vi "Example.vi"() -> ()   [LabVIEW 2020]
doc: "Demonstrate some of the aspect of the Firmata Protocol."
uses:
  FirmataClient/controls/PinModesListData.ctl
  FirmataClient/controls/PinModeData.ctl
  FirmataClient/controls/FirmataPinModes.ctl
  FirmataClient/controls/FGV-Mode.ctl
  FirmataClient.lvlib
panel:
  in  "Display Numbers As Decimal":bool
  in  "Send":bool
  in  "Stop":bool
  in  "Tab Control":T1(tab)
  out "Firmata Firmware Version GF":string caption="Firmata Firmware Version"
  out "Firmata Firmware Name GF":string caption="Firmata Firmware Name"
  out "IsValidSysex":bool
  out "FirmataFirmwareVersion":string
  out "IsValidReply":bool
  out "IsValidSysex 2":bool caption="IsValidSysex"
  out "Board Pins":T2[](array[typedef]) {"Index"."DigitalIndex" step=1 format="D%d"; "Index"."AnalogIndex" min=0.0 step=1.0 format="A%#.0g"}
  in  "Enable Reporting? SAPR":bool caption="Enable Reporting?"
  in  "Pin Index SAPR":u8 caption="Pin Index" format="%.0x"
  out "AnalogADCValues":u16[](array[numeric])
  in  "Pin Index GPS 2":u8 caption="Pin Index" format="%.0x"
  out "Pin Index GPS":u8 caption="Pin Index" format="%.0x"
  out "Pin State GPS":u64 caption="Pin State" format="%.0x"
  out "Pin Mode GPS":T4=enum."Extended.DHT" caption="Pin Mode"
  out "Analog Mappings":dbl[](array[numeric])
  in  "Enable Reporting?":bool
  in  "Port Index SDPR":u8 caption="Port Index" format="%.0x"
  out "PortValue":u16 format="%.0x"
  out "PortValueAsArray":bool[](array[boolean])
  out "Port Index 2":u8 format="%.0x"
  in  "Pin Index SPM":u8 caption="Pin Index" format="%.0x"
  in  "Pin Mode":T4
  in  "Pin State":bool
  in  "Pin Index SDP":u8 caption="Pin Index" format="%.0x"
  in  "Pin Value":u16 format="%.0x"
  in  "Pin Index":u8 format="%.0x"
  in  "Port State":bool[](array[boolean])
  in  "Port Index":u8 format="%.0x"
  in  "comport":refnum<visa-resource-name>="COM20"
  in  "baud rate":u32=57600
  out "Messages":string
  # "Set Board Comport and Baud Rate, Run the VI.\nWhen initialization is successful, select tab, read instructions and click on send.\n\nThis is a partial implementation of the Firmata protocol.\nFor more information, https://github.com/firmata/protocol/blob/master/protocol.md#message-types"
  # "Get the remote device/microcontroller to reset.\n\nClick on the \"Send Message\" button."
  # "Obtain the name of the sketch running on the remote device/microcontroller along with its version.\n\nClick on the \"Send Message\" button."
  # "Obtain the version of the sketch running on the remote device/microcontroller.\n\nClick on the \"Send Message\" button."
  # "In reporting mode, the remote device/microcontroller puts a message on the serial line everytime the value of the (input) line being reported on changes.\n\nPins are numbered from 0 to the total number of IO lines the microcontroller supports. One must then make sure to find the offset/index for the line.\n\nSet an index for the line to use,\nSet reporting to true or false.\n\nClick on the \"Send Message\" button."
  # "In reporting mode, the remote device/microcontroller puts a message on the serial line everytime the value of the (input) line being reported on changes.\n\nPins are numbered from 0 to the total number of IO lines the microcontroller supports. One must then make sure to find the offset/index for the line.\n\nSet an index for the line to use,\nSet reporting to true or false.\n\nClick on the \"Send Message\" button."
  # "In reporting mode, the remote device/microcontroller puts a message on the serial line everytime the value of the (input) line being reported on changes.\n\nPins are numbered from 0 to the total number of IO lines the microcontroller supports. One must then make sure to find the offset/index for the line.\n\nSet an index for the line to use,\nSet reporting to true or false.\n\nClick on the \"Send Message\" button."
  # "In reporting mode, the remote device/microcontroller puts a message on the serial line everytime the value of the (input) line being reported on changes.\n\nPins are numbered from 0 to the total number of IO lines the microcontroller supports. One must then make sure to find the offset/index for the line.\n\nSet an index for the line to use,\nSet reporting to true or false.\n\nClick on the \"Send Message\" button."
  # "The firmata protocol allows control of pin under various modes (digital input, output, analog input, pwm,...)\n\nPins are numbered from 0 to the total number of IO lines the microcontroller supports. One must then make sure to find the offset/index for the line.\n\nSet an index for the line to use,\nSet line new mode.\n\nClick on the \"Send Message\" button."
  # "In reporting mode, the remote device/microcontroller puts a message on the serial line everytime the value of the line being reported on changes.\n\nPins are numbered from 0 to the total number of IO lines the microcontroller supports. One must then make sure to find the offset/index for the line.\n\nSet an index for the line to use,\nSet reporting to true or false.\n\nClick on the \"Send Message\" button."
  # "An Analog message can convey the current value on the line or, if the line is configured as an analog output, the value for the DAC can be passed along. Typically this value is a 14bits value depending on the resolution of the pin\n\nPins are numbered from 0 to the total number of IO lines the microcontroller supports. One must then make sure to find the offset/index for the line.\n\nSet an index for the line to use,\nSet line value.\n\nClick on the \"Send Message\" button."
  # "Available pins are logically divided in ports of 8 bits each. Given the index of the pins to control, compute the index of the port (pinIndex / 8), and the offset of the pin within the port (pinIndex % 8) and set the required value.\n\nSet an index for the port to use,\nSet line states.\n\nClick on the \"Send Message\" button."
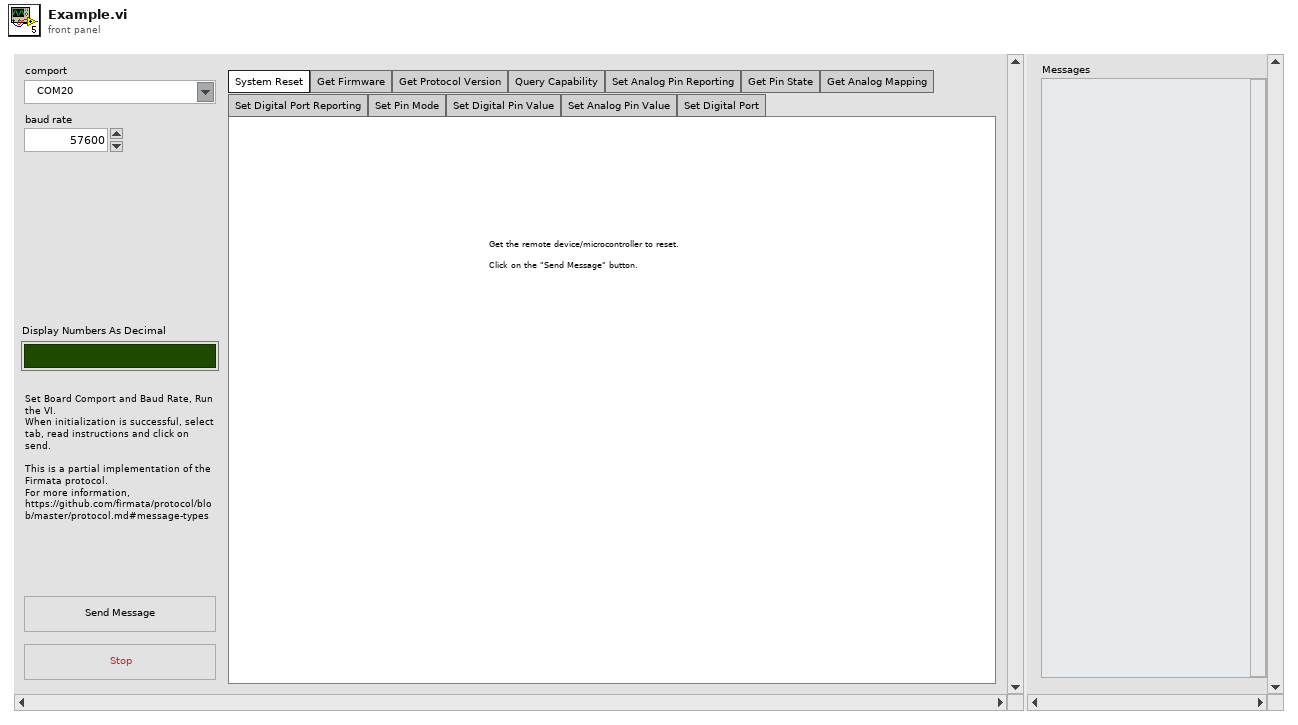
[diagram p1: front panel]
types:
  T1 = enum32{"System Reset", "Get Firmware", "Get Protocol Version", "Query Capability", "Set Analog Pin Reporting", "Get Pin State", "Get Analog Mapping", "Set Digital Port Reporting", "Set Pin Mode", "Set Digital Pin Value", "Set Analog Pin Value", "Set Digital Port"}
  T2 = typedef "FirmataClient.lvlib/PinModesListData.ctl" = cluster{"DigitalInputMode":T3, "DigitalOutputMode":T3, "AnalogInputMode":T3, "PWMMode":T3, "ServoMode":T3, "ShiftMode":T3, "I2CMode":T3, "OneWireMode":T3, "StepperMode":T3, "EncoderMode":T3, "SerialMode":T3, "InputPullupMode":T3, "Ext.SPIMode":T3, "Ext.SonarMode":T3, "Ext.ToneMode":T3, "Ext.DHTMode":T3, "Index":cluster{"DigitalIndex":u16, "AnalogIndex":dbl}}
  T3 = typedef "FirmataClient.lvlib/PinModeData.ctl" = cluster{"Resolution":u8, "btn":bool, "PinMode":T4}
  T4 = typedef "FirmataClient.lvlib/FirmataPinModes.ctl" = enum16{"DigitalInput", "DigitalOutput", "AnalogInput", "PWM", "Servo", "Shift", "I2C", "OneWire", "Stepper", "Encoder", "Serial", "InputPullup", "Extended.SPI", "Extended.Sonar", "Extended.Tone", "Extended.DHT"}
  T5 = typedef "FirmataClient.lvlib/FGV-Mode.ctl" = enum16{"Load Comport", "Load Board Capabilities", "Read"}
  T6 = typedef "FirmataClient.lvlib/FirmataProtocolConstants.ctl" = u16
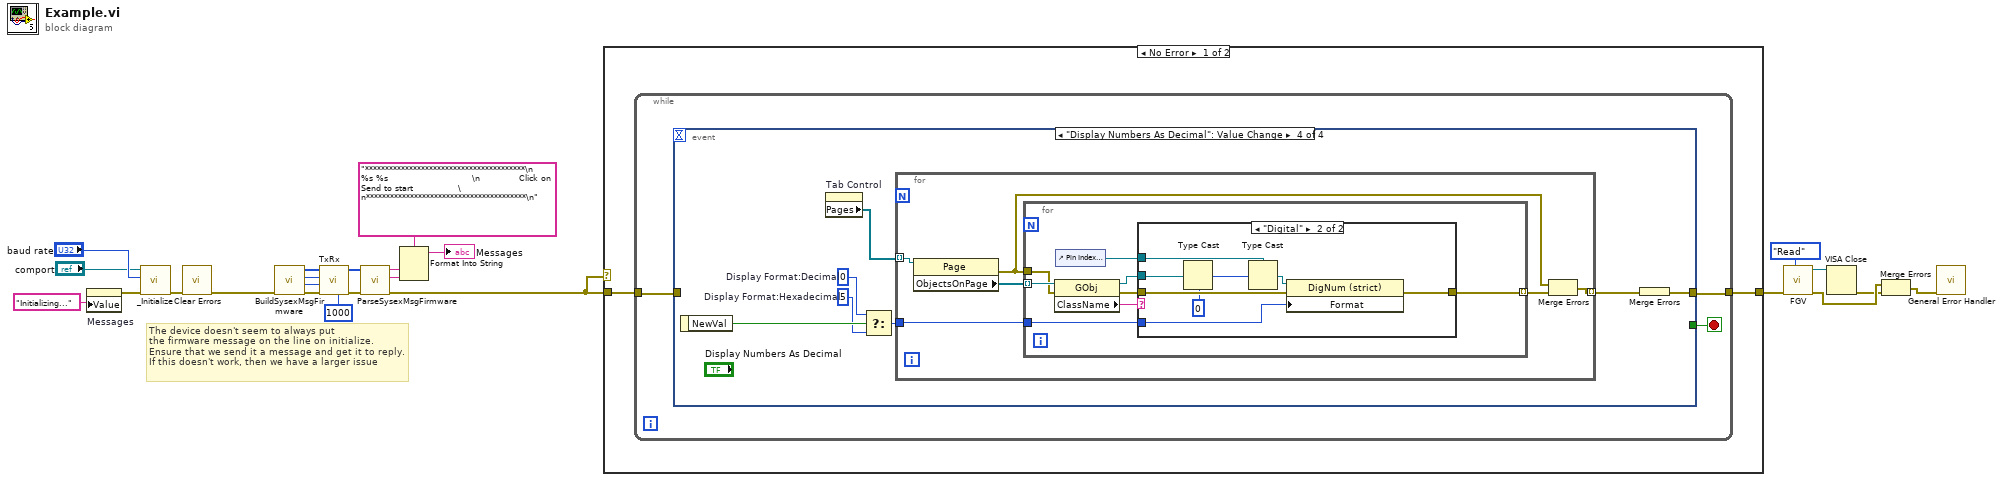
[diagram p0: block diagram]
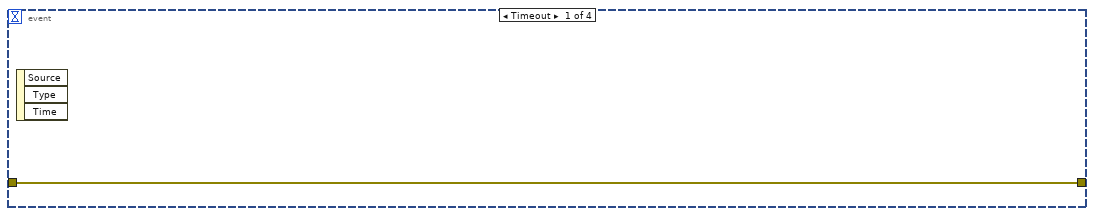
[diagram p2: hidden frame]
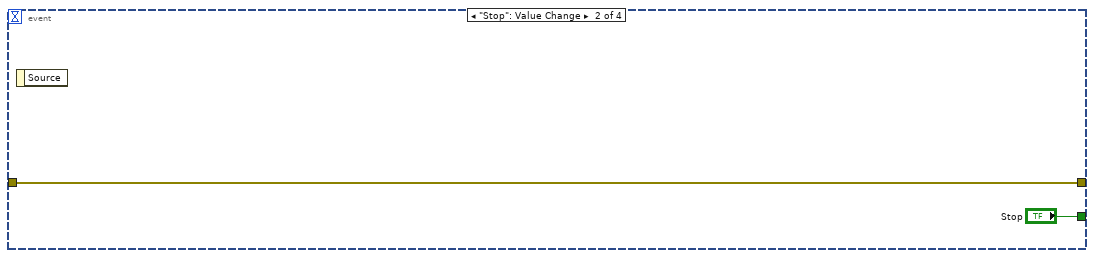
[diagram p3: hidden frame]
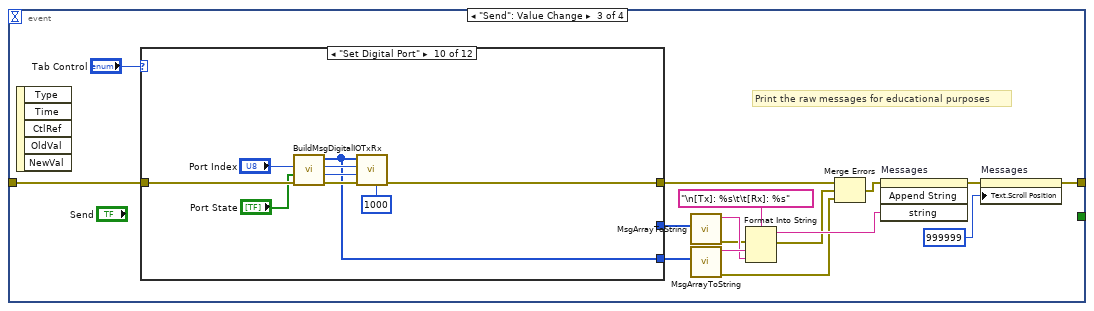
[diagram p4: hidden frame]
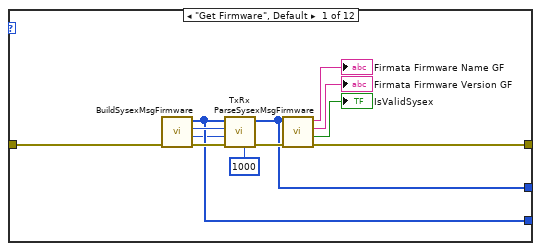
[diagram p5: hidden frame]
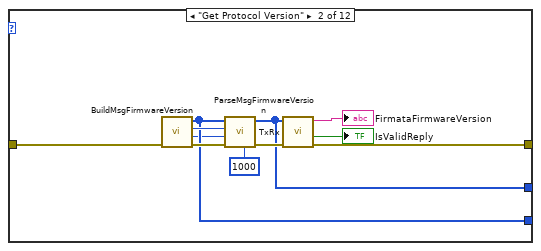
[diagram p6: hidden frame]
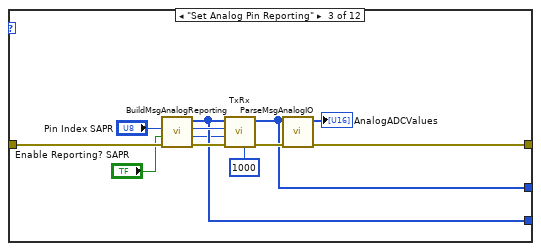
[diagram p7: hidden frame]
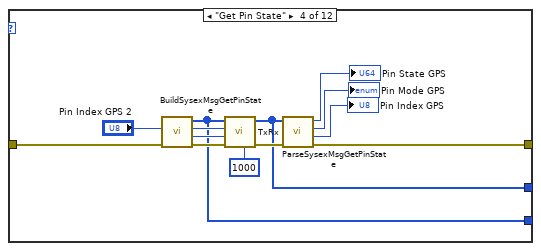
[diagram p8: hidden frame]
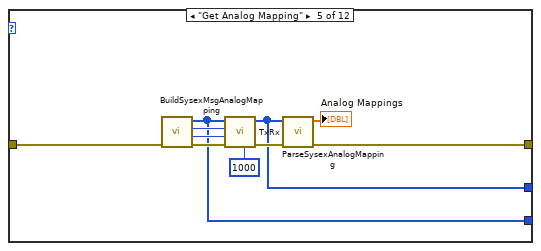
[diagram p9: hidden frame]
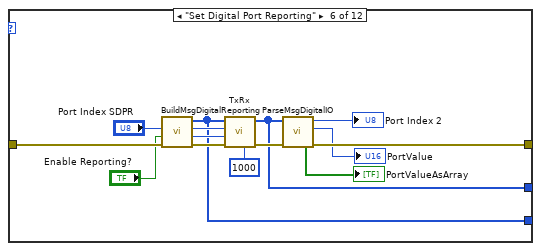
[diagram p10: hidden frame]
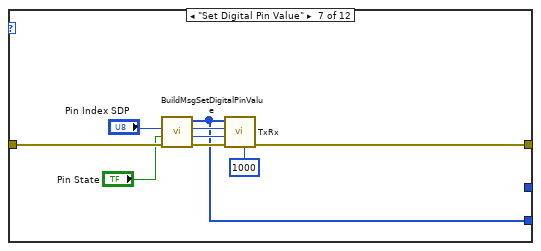
[diagram p11: hidden frame]
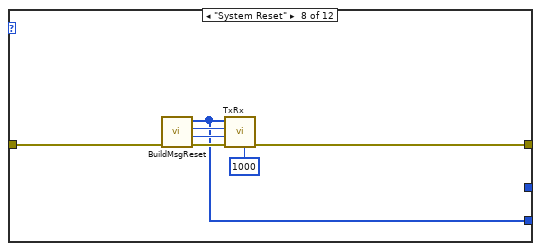
[diagram p12: hidden frame]
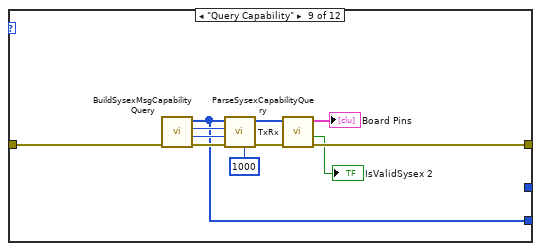
[diagram p13: hidden frame]
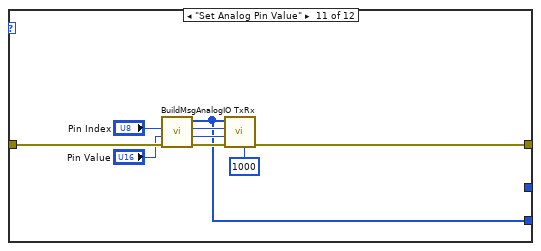
[diagram p14: hidden frame]
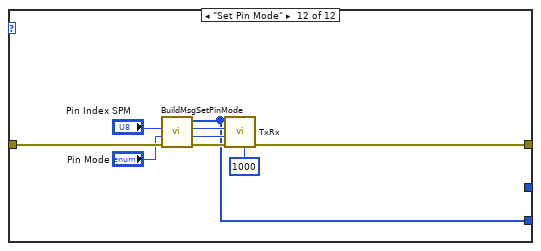
[diagram p15: hidden frame]
diagram:
  # "The device doesn't seem to always put \nthe firmware message on the line on initialize.\nEnsure that we send it a message and get it to reply.\nIf this doesn't work, then we have a larger issue"
  n1 = property on="Messages" class="Str"("Value"="Initializing..." ("Messages")) -> (error out=w19:errorcluster)  [unwired: 2 in, 1 out]
  n2 = call "_Initialize.vi"("error in"=w19, "baud rate"="baud rate", "comport"="comport") -> ("error out"=w15:errorcluster)  [unwired: 4 in, 4 out]
  n3 = call <vilib>:"Clear Errors.vi"("error in (no error)"=w15) -> ("error out"=w4:errorcluster)  [unwired: 5 in, 1 out]
  n4 = call "BuildSysexMsgFirmware.vi"("error in"=w4) -> ("error out"=w10:errorcluster, "ReplyLength"=w8:i32, "ReplyFirstByte"=w7:T6, "GetFirmwareMessage"=w6:u8[])  [unwired: 7 in]
  n5 = call "TxRx.vi"("Timeout"=u32 1000, "error in"=w10, "Expected Reply Length"=w8, "ReplyFirstByte"=w7, "MessageToSend"=w6) -> ("error out"=w11:errorcluster, "ReceivedMessage"=w5:u8[])  [unwired: 2 in, 3 out]
  n6 = call "ParseSysexMsgFirmware.vi"("error in"=w11, "Sysex Message"=w5) -> ("error out"=w3:errorcluster, "FirmataFirmwareVersion"=w2:string, "FirmataFirmwareName"=w1:string)  [unwired: 6 in, 1 out]
  n7 = Format Into String(format string="****************************************\n         %s %s                            \n             Click on Send to start               \n****************************************\n", w1, w2) -> (resulting string=→"Messages":string)  [unwired: 2 in, 1 out]
  n8 = case shown="No Error" w3 {
    tunnel: [w26 w204] -> w22
    tunnel: w3 -> [w25 w204]
    frame No Error {
      n9 = while {
        tunnel: [w28] -> w26
        tunnel: w25 -> [w27]
        stop <- w29 stop-if-true
        n10 = event shown="[3] \"Display Numbers As Decimal\": Value Change" {
          selector: _ -> [_ _ _ _]
          dyn-events: _ -> [_ _ _ _]
          timeout: _ -> [_ _ _ _]
          tunnel: [_ "Stop" _ _] -> w29
          tunnel: [w30 w31 w45 w175] -> w28
          tunnel: w27 -> [w30 w31 w48 _]
          event Timeout {
            n11 = event-data() -> ()  [unwired: 1 in, 3 out]
          }
          event "Stop": Value Change {
            n12 = event-data() -> ()  [unwired: 1 in, 1 out]
          }
          event "Send": Value Change {
            # "Print the raw messages for educational purposes"
            n13 = event-data() -> ()  [unwired: 1 in, 5 out]
            n14 = case shown="\"Set Digital Port\"" "Tab Control" {
              tunnel: [w57 w68 w80 w93 w103 w117 w127 w134 w144 w154 w163 w172] -> w34
              tunnel: w48 -> [w60 w71 w83 w96 w106 w120 w129 w136 w147 w156 w165 w174]
              tunnel: [w51 w64 w76 w84 w97 w112 w121 w130 w138 w148 w157 w168] -> w38
              tunnel: [w49 w62 w75 w85 w98 w111 _ _ _ _ _ _] -> w39
              frame "Get Firmware", Default {
                n15 = call "BuildSysexMsgFirmware.vi"("error in"=w60) -> ("error out"=w59:errorcluster, "ReplyLength"=w50:i32, "ReplyFirstByte"=w55:T6, "GetFirmwareMessage"=w51:u8[])  [unwired: 7 in]
                n16 = call "TxRx.vi"("Timeout"=u32 1000, "error in"=w59, "Expected Reply Length"=w50, "ReplyFirstByte"=w55, "MessageToSend"=w51) -> ("error out"=w58:errorcluster, "ReceivedMessage"=w49:u8[])  [unwired: 2 in, 3 out]
                n17 = call "ParseSysexMsgFirmware.vi"("error in"=w58, "Sysex Message"=w49) -> ("error out"=w57:errorcluster, "IsValidSysex"=→"IsValidSysex":bool, "FirmataFirmwareVersion"=→"Firmata Firmware Version GF":string, "FirmataFirmwareName"=→"Firmata Firmware Name GF":string)  [unwired: 6 in]
              }
              frame "Get Protocol Version" {
                n18 = call "BuildMsgFirmwareVersion.vi"("error in"=w71) -> ("error out"=w70:errorcluster, "ReplyLength"=w61:i32, "ReplyFirstByte"=w66:T6, "GetFirmwareMessage"=w64:u8[])  [unwired: 7 in]
                n19 = call "TxRx.vi"("Timeout"=u32 1000, "error in"=w70, "Expected Reply Length"=w61, "ReplyFirstByte"=w66, "MessageToSend"=w64) -> ("error out"=w69:errorcluster, "ReceivedMessage"=w62:u8[])  [unwired: 2 in, 3 out]
                n20 = call "ParseMsgFirmwareVersion.vi"("error in"=w69, "Sysex Message"=w62) -> ("error out"=w68:errorcluster, "IsValidReply"=→"IsValidReply":bool, "FirmataFirmwareVersion"=→"FirmataFirmwareVersion":string)  [unwired: 7 in]
              }
              frame "Set Analog Pin Reporting" {
                n21 = call "BuildMsgAnalogReporting.vi"("error in"=w83, "Enable Reporting?"="Enable Reporting? SAPR", "Pin Index"="Pin Index SAPR") -> ("error out"=w82:errorcluster, "ReplyLength"=w74:i32, "ReplyFirstByte"=w78:T6, "AnalogReportingMessage"=w76:u8[])  [unwired: 5 in]
                n22 = call "TxRx.vi"("Timeout"=u32 1000, "error in"=w82, "Expected Reply Length"=w74, "ReplyFirstByte"=w78, "MessageToSend"=w76) -> ("error out"=w81:errorcluster, "ReceivedMessage"=w75:u8[])  [unwired: 2 in, 3 out]
                n23 = call "ParseMsgAnalogIO.vi"("error in"=w81, "Sysex Message"=w75) -> ("error out"=w80:errorcluster, "AnalogADCValues"=→"AnalogADCValues":u16[])  [unwired: 8 in]
              }
              frame "Get Pin State" {
                n24 = call "BuildSysexMsgGetPinState.vi"("error in"=w96, "Pin Index"="Pin Index GPS 2") -> ("error out"=w95:errorcluster, "ReplyLength"=w87:i32, "ReplyFirstByte"=w91:T6, "GetPinStateMessage"=w84:u8[])  [unwired: 6 in]
                n25 = call "TxRx.vi"("Timeout"=u32 1000, "error in"=w95, "Expected Reply Length"=w87, "ReplyFirstByte"=w91, "MessageToSend"=w84) -> ("error out"=w94:errorcluster, "ReceivedMessage"=w85:u8[])  [unwired: 2 in, 3 out]
                n26 = call "ParseSysexMsgGetPinState.vi"("error in"=w94, "Sysex Message"=w85) -> ("error out"=w93:errorcluster, "Pin Index"=→"Pin Index GPS":u8, "Pin Mode"=→"Pin Mode GPS":T4, "Pin State"=→"Pin State GPS":u64)  [unwired: 6 in]
              }
              frame "Get Analog Mapping" {
                n27 = call "BuildSysexMsgAnalogMapping.vi"("error in"=w106) -> ("error out"=w105:errorcluster, "ReplyLength"=w100:i32, "ReplyFirstByte"=w101:T6, "GetAnalogMappingMessage"=w97:u8[])  [unwired: 7 in]
                n28 = call "TxRx.vi"("Timeout"=u32 1000, "error in"=w105, "Expected Reply Length"=w100, "ReplyFirstByte"=w101, "MessageToSend"=w97) -> ("error out"=w104:errorcluster, "ReceivedMessage"=w98:u8[])  [unwired: 2 in, 3 out]
                n29 = call "ParseSysexAnalogMapping.vi"("error in"=w104, "Sysex Message"=w98) -> ("error out"=w103:errorcluster, "AnalogChannels"=→"Analog Mappings":dbl[])  [unwired: 7 in, 1 out]
              }
              frame "Set Digital Port Reporting" {
                n30 = call "BuildMsgDigitalReporting.vi"("error in"=w120, "Enable Reporting?"="Enable Reporting?", "Port Index"="Port Index SDPR") -> ("error out"=w119:errorcluster, "ReplyLength"=w113:i32, "ReplyFirstByte"=w115:T6, "DigitalReportingMessage"=w112:u8[])  [unwired: 5 in]
                n31 = call "TxRx.vi"("Timeout"=u32 1000, "error in"=w119, "Expected Reply Length"=w113, "ReplyFirstByte"=w115, "MessageToSend"=w112) -> ("error out"=w118:errorcluster, "ReceivedMessage"=w111:u8[])  [unwired: 2 in, 3 out]
                n32 = call "ParseMsgDigitalIO.vi"("error in"=w118, "Sysex Message"=w111) -> ("error out"=w117:errorcluster, "PortValue"=→"PortValue":u16, "Port Index"=→"Port Index 2":u8, "PortValueAsArray"=→"PortValueAsArray":bool[])  [unwired: 6 in]
              }
              frame "Set Digital Pin Value" {
                n33 = call "BuildMsgSetDigitalPinValue.vi"("error in"=w129, "Pin Value"="Pin State", "Pin Index"="Pin Index SDP") -> ("error out"=w128:errorcluster, "ReplyLength"=w124:i32, "ReplyFirstByte"=w125:T6, "DigitalPinValueMessage"=w121:u8[])  [unwired: 5 in]
                n34 = call "TxRx.vi"("Timeout"=u32 1000, "error in"=w128, "Expected Reply Length"=w124, "ReplyFirstByte"=w125, "MessageToSend"=w121) -> ("error out"=w127:errorcluster)  [unwired: 2 in, 4 out]
              }
              frame "System Reset" {
                n35 = call "BuildMsgReset.vi"("error in"=w136) -> ("error out"=w135:errorcluster, "ReplyLength"=w131:i32, "ReplyFirstByte"=w132:T6, "ResetMessage"=w130:u8[])  [unwired: 7 in]
                n36 = call "TxRx.vi"("Timeout"=u32 1000, "error in"=w135, "Expected Reply Length"=w131, "ReplyFirstByte"=w132, "MessageToSend"=w130) -> ("error out"=w134:errorcluster)  [unwired: 2 in, 4 out]
              }
              frame "Query Capability" {
                n37 = call "BuildSysexMsgCapabilityQuery.vi"("error in"=w147) -> ("error out"=w146:errorcluster, "ReplyLength"=w140:i32, "ReplyFirstByte"=w142:T6, "GetCapabilitiesMessage"=w138:u8[])  [unwired: 7 in]
                n38 = call "TxRx.vi"("Timeout"=u32 1000, "error in"=w146, "Expected Reply Length"=w140, "ReplyFirstByte"=w142, "MessageToSend"=w138) -> ("error out"=w145:errorcluster, "ReceivedMessage"=w139:u8[])  [unwired: 2 in, 3 out]
                n39 = call "ParseSysexCapabilityQuery.vi"("error in"=w145, "Sysex Message"=w139) -> ("error out"=w144:errorcluster, "IsValidSysex"=→"IsValidSysex 2":bool, "Board Pins"=→"Board Pins":T2[])  [unwired: 7 in]
              }
              frame "Set Digital Port" {
                n40 = call "BuildMsgDigitalIO.vi"("error in"=w156, "Port"="Port State", "Port Index"="Port Index") -> ("error out"=w155:errorcluster, "ReplyLength"=w151:i32, "ReplyFirstByte"=w152:T6, "DigitalIOMessage"=w148:u8[])  [unwired: 5 in]
                n41 = call "TxRx.vi"("Timeout"=u32 1000, "error in"=w155, "Expected Reply Length"=w151, "ReplyFirstByte"=w152, "MessageToSend"=w148) -> ("error out"=w154:errorcluster)  [unwired: 2 in, 4 out]
              }
              frame "Set Analog Pin Value" {
                n42 = call "BuildMsgAnalogIO.vi"("error in"=w165, "Pin Value"="Pin Value", "Pin Index"="Pin Index") -> ("error out"=w164:errorcluster, "ReplyLength"=w160:i32, "ReplyFirstByte"=w161:T6, "AnalogIOMessage"=w157:u8[])  [unwired: 5 in]
                n43 = call "TxRx.vi"("Timeout"=u32 1000, "error in"=w164, "Expected Reply Length"=w160, "ReplyFirstByte"=w161, "MessageToSend"=w157) -> ("error out"=w163:errorcluster)  [unwired: 2 in, 4 out]
              }
              frame "Set Pin Mode" {
                n44 = call "BuildMsgSetPinMode.vi"("error in"=w174, "Pin Mode"="Pin Mode", "Pin Index"="Pin Index SPM") -> ("error out"=w173:errorcluster, "ReplyLength"=w169:i32, "ReplyFirstByte"=w170:T6, "SetPinModeMessage"=w168:u8[])  [unwired: 5 in]
                n45 = call "TxRx.vi"("Timeout"=u32 1000, "error in"=w173, "Expected Reply Length"=w169, "ReplyFirstByte"=w170, "MessageToSend"=w168) -> ("error out"=w172:errorcluster)  [unwired: 2 in, 4 out]
              }
            }
            n46 = call "MsgArrayToString.vi"("Message In"=w39) -> ("error out"=w37:errorcluster, "Message Out"=w42:string)  [unwired: 9 in]
            n47 = call "MsgArrayToString.vi"("Message In"=w38) -> ("error out"=w36:errorcluster, "Message Out"=w43:string)  [unwired: 9 in]
            n48 = Format Into String(format string="\n[Tx]: %s\t\t[Rx]: %s", error in=w37, w43, w42) -> (resulting string=w40:string, error out=w35:errorcluster)  [unwired: 1 in]
            n49 = Merge Errors(w34, w35, w36) -> (w33:errorcluster)
            n50 = invoke on="Messages" class="Str" method="Append String"(error in=w33, "string"=w40) -> (error out=w46:errorcluster)  [unwired: 2 in, 3 out]
            n51 = property on="Messages" class="Str"(error in=w46, "Text.Scroll Position"=u32 999999) -> (error out=w45:errorcluster)  [unwired: 1 in, 1 out]
          }
          event "Display Numbers As Decimal": Value Change {
            w178 = u8 0  # Display Format:Decimal
            w179 = u8 5  # Display Format:Hexadecimal
            n52 = event-data() -> ("NewVal"=w180:bool)  [unwired: 1 in]
            n53 = property on="Tab Control" class="TabCtl (strict)"() -> ("Pages"=w181:refnum<vi>[])  [unwired: 2 in, 2 out]
            n54 = Select(t=w178, s=w180, f=w179) -> (s? t:f=w177:u8)
            n55 = for {
              tunnel: w181 -> [w187] mode=indexing
              tunnel: w177 -> [w185]
              tunnel: [w183] -> w176 mode=indexing
              n56 = property class="Page"(reference=w187) -> (error out=w182:errorcluster, "ObjectsOnPage"=w186:refnum<vi>[])  [unwired: 1 in, 1 out]
              n57 = for {
                tunnel: w186 -> [w195] mode=indexing
                tunnel: w185 -> [w191]
                tunnel: [w190] -> w184 mode=indexing
                tunnel: w182 -> [w189]
                n58 = property class="GObj"(reference=w195, error in=w189) -> (reference out=w193:refnum<vi>, error out=w188:errorcluster, "ClassName"=w194:string)
                n59 = control-ref of="Pin Index SPM"() -> (w192:refnum<vi>)
                n60 = case shown="\"Digital\"" w194 {
                  tunnel: w193 -> [_ w198]
                  tunnel: w192 -> [_ w203]
                  tunnel: w191 -> [_ w201]
                  tunnel: [_ w200] -> w190
                  tunnel: w188 -> [_ w199]
                  frame "False", Default {
                  }
                  frame "Digital" {
                    n61 = Type Cast(type=0, x=w198) -> (*(type *) &x=w197:i32)
                    n62 = Type Cast(type=w203, x=w197) -> (*(type *) &x=w202:refnum<vi>)
                    n63 = property class="DigNum (strict)"(reference=w202, error in=w199, "Format"=w201) -> (error out=w200:errorcluster)  [unwired: 1 out]
                  }
                }
              }
              n64 = Merge Errors(w182, w184) -> (w183:errorcluster)
            }
            n65 = Merge Errors(w176) -> (w175:errorcluster)
          }
        }
      }
    }
    frame Error {
    }
  }
  n66 = call "FGV.vi"("Mode"=FGV-Mode."Read", "error in"=w22) -> ("error out"=w14:errorcluster, "comport out"=w21:refnum<visa-resource-name>)  [unwired: 7 in, 1 out]
  n67 = VISA Close(VISA resource name=w21) -> (error out=w13:errorcluster)  [unwired: 1 in]
  n68 = Merge Errors(w14, w13) -> (w12:errorcluster)
  n69 = call <vilib>:"General Error Handler.vi"("error in (no error)"=w12) -> ()  [unwired: 10 in, 5 out]
